vi "SavingThread.vi"(8 "error in (no error)":errorcluster, 11 "Application Data":T1) -> (0 "error out":errorcluster)   [LabVIEW 2019]
uses:
  Typedefs/#cluster_ApplicationData.ctl
  Typedefs/Acquisition Thread/#cluster_AcqQueueData.ctl
  Typedefs/Acquisition Thread/#enum_AcquisitionTask.ctl
  Typedefs/Saving Thread/#cluster_SavingQueueData.ctl
  Typedefs/Saving Thread/#enum_SavingTask.ctl
  Typedefs/Saving Thread/#cluster_SavingThreadData.ctl
  LowLevelError.vi
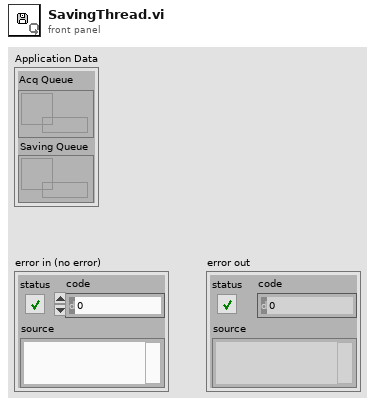
[diagram p1: front panel]
types:
  T1 = typedef "#cluster_ApplicationData.ctl" = cluster{"Acq Queue":refnum<queue>, "Saving Queue":refnum<queue>}
  T2 = typedef "#cluster_SavingThreadData.ctl" = cluster{"Measurement Directory":path, "File ref":refnum<k34>, "File opened?":bool}
  T3 = typedef "#cluster_SavingQueueData.ctl" = cluster{"Task":T4, "Data":variant}
  T4 = typedef "#enum_SavingTask.ctl" = enum16{"Set directory", "Save", "Stop", "Close"}
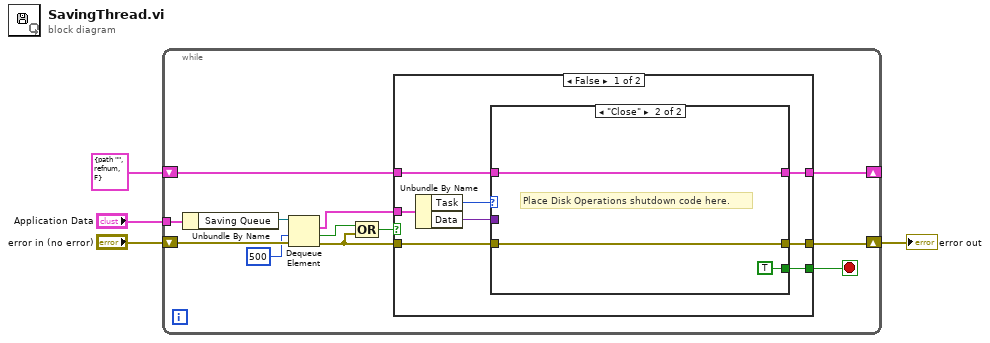
[diagram p0: block diagram]
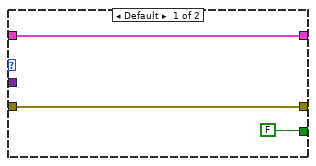
[diagram p2: hidden frame]
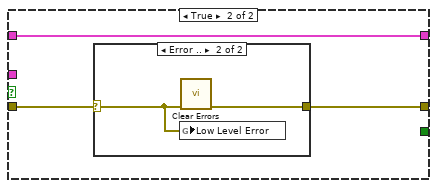
[diagram p3: hidden frame]
diagram:
  n1 = while {
    tunnel: "Application Data" -> [w11]
    shift-right: [w6] -> w2
    shift-left: "error in (no error)" -> [w16]
    shift-right: [w5] -> _
    shift-left: T2 {"Measurement Directory"=path "", "File ref"=refnum, "File opened?"=FALSE} ("Saving Thread Data") -> [w12]
    stop <- w13 stop-if-true
    n2 = Unbundle By Name(w11) -> ("Saving Queue"=w15:refnum<queue>)
    n3 = Dequeue Element(queue=w15, timeout in ms (-1)=500, error in (no error)=w16) -> (element=w14:T3, timed out?=w9:bool, error out=w7:errorcluster)  [unwired: 1 out]
    n4 = Compound Arithmetic op=OR(w9, w7) -> (w8:bool)
    n5 = case shown="False" w8 {
      tunnel: w14 -> [w24 _]
      tunnel: w7 -> [w21 w32]
      tunnel: [w20 _] -> w13
      tunnel: w12 -> [w19 w33]
      tunnel: [w18 w33] -> w5
      tunnel: [w17 w31] -> w6
      frame False {
        n6 = Unbundle By Name(w24) -> ("Task"=w23:T4, "Data"=w22:variant)
        n7 = case shown="\"Close\"" w23 {
          tunnel: w22 -> [_ _]
          tunnel: w21 -> [w26 w29]
          tunnel: [w27 w30] -> w18
          tunnel: [FALSE TRUE] -> w20
          tunnel: w19 -> [w27 w30]
          tunnel: [w26 w29] -> w17
          frame Default {
          }
          frame "Close" {
            # "Place Disk Operations shutdown code here."
          }
        }
      }
      frame True {
        n8 = case shown="Error .." w32 {
          selector: w32 -> [w34 w35]
          tunnel: [w34 w36] -> w31
          frame No Error {
          }
          frame Error {
            n9 = global write "LowLevelError.vi" "Low Level Error"(w35) -> ()
            n10 = call <vilib>:"Clear Errors.vi"("error in (no error)"=w35) -> ("error out"=w36:errorcluster)  [unwired: 5 in, 1 out]
          }
        }
      }
    }
  }
  "error out" <- w2
